vi "Write Interpolate color.vi"(5 "Interpolate color":bool, 9 "ColorScale in":refnum<class "ColorScale.lvclass">) -> (3 "ColorScale out":refnum<class "ColorScale.lvclass">)   [LabVIEW 2014, in "Raspberry Pi Compatible Compiler for LabVIEW.lvlib" / "ColorScale.lvclass"]
uses:
  ColorScale.lvclass
  ColorScale.lvclass/ColorScale.ctl
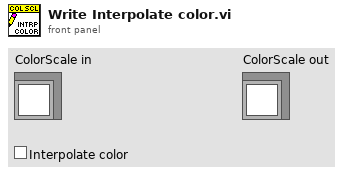
[diagram p1: front panel]
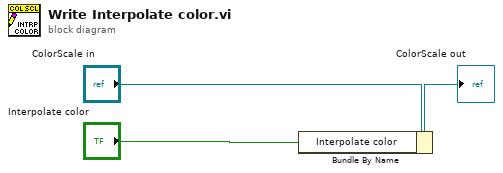
[diagram p0: block diagram]
diagram:
  n1 = Bundle By Name(cluster="ColorScale in", "Interpolate color"="Interpolate color") -> (→"ColorScale out":refnum<class "ColorScale.lvclass">)
